vi "Send Goal Info.vi"(1 "Target Info":T2(array[cluster])) -> ()   [LabVIEW 2013]
uses:
  TargetType.ctl
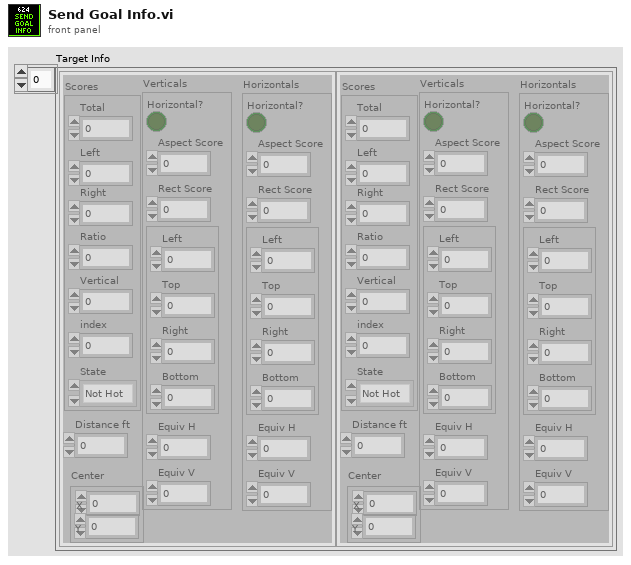
[diagram p1: front panel]
types:
  T1 = typedef "TargetType.ctl" = enum16{"Not Hot", "Hot"}
  T2 = cluster{"Scores":cluster{"Total":dbl, "Left":dbl, "Right":dbl, "Ratio":dbl, "Vertical":dbl, "index":i32, "State":T1}, "Verticals":cluster{"Horizontal?":bool, "Aspect Score":dbl, "Rect Score":dbl, cluster{"Left":dbl, "Top":dbl, "Right":dbl, "Bottom":dbl}, "Equiv H":dbl, "Equiv V":dbl}, "Horizontals":cluster{"Horizontal?":bool, "Aspect Score":dbl, "Rect Score":dbl, cluster{"Left":dbl, "Top":dbl, "Right":dbl, "Bottom":dbl}, "Equiv H":dbl, "Equiv V":dbl}, "Distance ft":dbl, "Center":cluster{"X":dbl, "Y":dbl}}[]
  T3 = cluster{"Scores":cluster{"Total":dbl, "Left":dbl, "Right":dbl, "Ratio":dbl, "Vertical":dbl, "index":i32, "State":T1}, "Verticals":cluster{"Horizontal?":bool, "Aspect Score":dbl, "Rect Score":dbl, cluster{"Left":dbl, "Top":dbl, "Right":dbl, "Bottom":dbl}, "Equiv H":dbl, "Equiv V":dbl}, "Horizontals":cluster{"Horizontal?":bool, "Aspect Score":dbl, "Rect Score":dbl, cluster{"Left":dbl, "Top":dbl, "Right":dbl, "Bottom":dbl}, "Equiv H":dbl, "Equiv V":dbl}, "Distance ft":dbl, "Center":cluster{"X":dbl, "Y":dbl}}
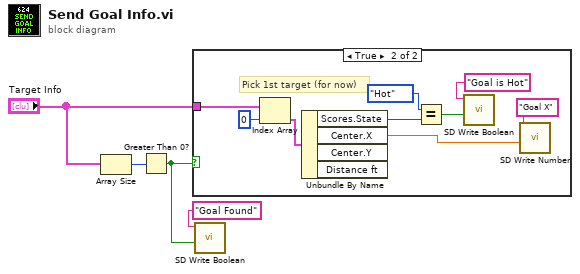
[diagram p0: block diagram]
diagram:
  n1 = Array Size(array="Target Info") -> (size(s)=w4:i32)
  n2 = Greater Than 0?(x=w4) -> (x > 0?=w1:bool)
  n3 = case shown="True" w1 {
    tunnel: "Target Info" -> [_ w13]
    frame False {
    }
    frame True {
      # "Pick 1st target (for now)"
      n4 = Index Array(array=w13, index=0) -> (element=w11:T3)
      n5 = Unbundle By Name(w11) -> ("Scores.State"=w10:T1, "Center.X"=w7:dbl)  [unwired: 2 out]
      n6 = Equal?(x=TargetType."Hot", y=w10) -> (x = y?=w6:bool)
      n7 = call <vilib>:"SD Write Boolean.vi"("Boolean"=w6, "Name"="Goal is Hot") -> ()  [unwired: 8 in, 2 out]
      n8 = call <vilib>:"SD Write Number.vi"("Numeric"=w7, "Name"="Goal X") -> ()  [unwired: 8 in, 2 out]
    }
  }
  n9 = call <vilib>:"SD Write Boolean.vi"("Boolean"=w1, "Name"="Goal Found") -> ()  [unwired: 8 in, 2 out]
